vi "setUp.vi"(8 "error in (no error)":errorcluster, 11 "reference in":refnum<class "Host API Tests.lvclass">) -> (0 "error out":errorcluster, 3 "reference out":refnum<class "Host API Tests.lvclass">)   [LabVIEW 2018, in "Host API Tests.lvclass"]
doc: "setUp runs prior to the test method during test execution. Use this method to initialize any object data required by your tests."
uses:
  Host API Tests.lvclass
  <vilib>/addons/_JKI Toolkits/VI Tester/TestCase.llb/TestCase.lvclass
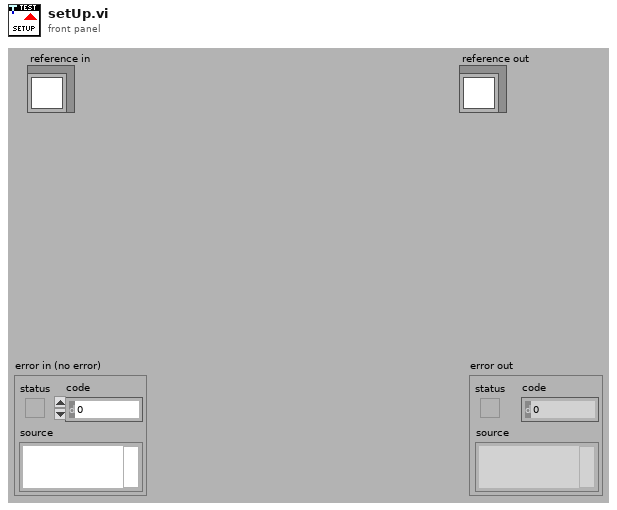
[diagram p1: front panel]
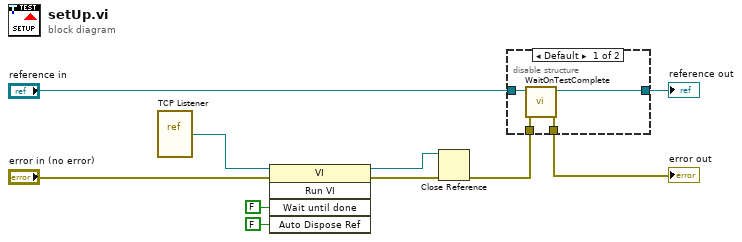
[diagram p0: block diagram]
diagram:
  n1 = vi-ref "TCP Listener.vi"() -> (w10:refnum<vi>)
  n2 = invoke class="VI" method="Run VI"(reference=w10, error in="error in (no error)", "Wait until done"=FALSE ("Wait Until Done"), "Auto Dispose Ref"=FALSE ("Auto Dispose Reference")) -> (reference out=w9:refnum<vi>, error out=w8:errorcluster)  [unwired: 1 in, 3 out]
  n3 = Close Reference(reference=w9, error in (no error)=w8) -> (error out=w7:errorcluster)
  n4 = disable-structure shown="Default" {
    disable-tunnel: w7 -> [w14 w15]
    disable-tunnel: [w13 w15] -> w1
    disable-tunnel: [w12 w16] -> w3
    disable-tunnel: "reference in" -> [w11 w16]
    frame condition #0 (active) {
      n5 = call <vilib>:"WaitOnTestComplete.vi"("error in (no error)"=w14, "TestCase in"=w11) -> ("error out"=w13:errorcluster, "TestCase out"=w12:refnum<class "Host API Tests.lvclass">)  [unwired: 8 in]
    }
    frame condition #1 {
    }
  }
  "error out" <- w1
  "reference out" <- w3
